vi "Update.vi"(8 "error in":errorcluster, 10 "object ref in":T1, 11 "Multi Column Listbox in":refnum<class "Multi Column Listbox.lvclass">) -> (0 "error out":errorcluster, 2 "object ref out":T1, 3 "Multi Column Listbox out":refnum<class "Multi Column Listbox.lvclass">)   [LabVIEW 2013, in "Table Manager.lvlib" / "Multi Column Listbox.lvclass"]
doc: "Updates the strings displayed in the MCLB."
uses:
  Multi Column Listbox.lvclass
  Table Manager/object ref.ctl
  Configuration Editor/Classes/Engine Parent/Engine Parent Editor Node.lvclass
  Configuration Editor/Classes/Module editor node/module editor node.lvclass
  Multi Column Listbox.lvclass/Multi Column Listbox.ctl
  Table Manager/Table Manager.lvclass/Table Manager.ctl
  Read Listbox.vi
  Table Manager/Read Index.vi
  Table Manager/Table Manager.lvclass
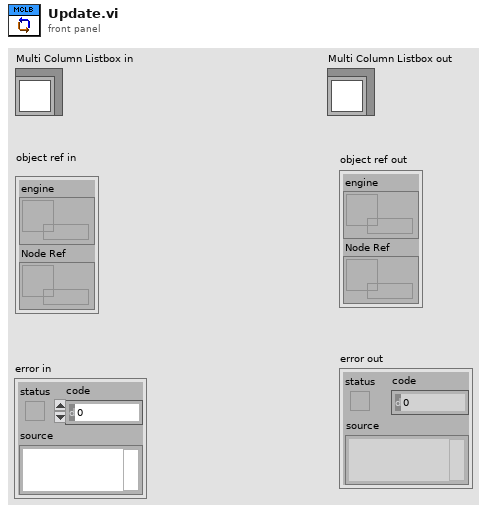
[diagram p1: front panel]
types:
  T1 = typedef "Table Manager.lvlib/Table Manager.lvclass/object ref.ctl" = cluster{"engine":refnum<data-value>, "Node Ref":refnum<data-value>}
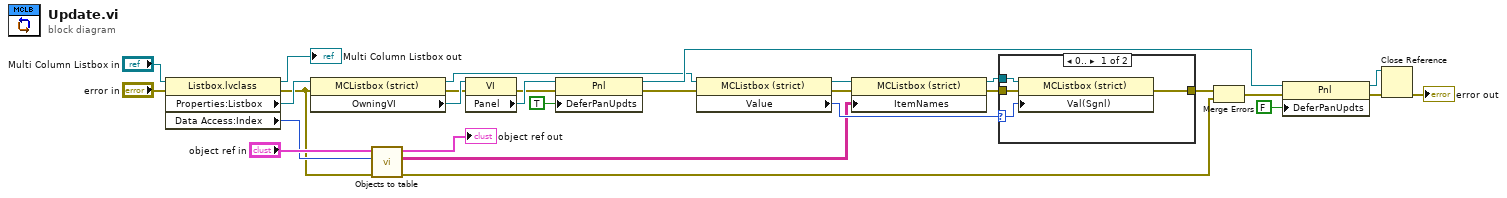
[diagram p0: block diagram]
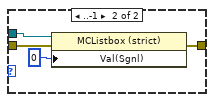
[diagram p2: hidden frame]
diagram:
  n1 = property class="Listbox.lvclass"(reference="Multi Column Listbox in", error in="error in") -> (reference out=→"Multi Column Listbox out":refnum<class "Multi Column Listbox.lvclass">, error out=w1:errorcluster, "Properties:Listbox"=w5:refnum<vi>, "Data Access:Index"=w6:i32)
  n2 = property class="MCListbox (strict)"(reference=w5, error in=w1) -> (reference out=w23:refnum<vi>, error out=w21:errorcluster, "OwningVI"=w22:refnum<vi>)
  n3 = call "Objects to table.vi"("error in (no error)"=w1, "Table Index"=w6, "object ref in"="object ref in") -> ("error out"=w9:errorcluster, "table"=w12:string[][], "object ref out"=→"object ref out":T1)  [unwired: 6 in]
  n4 = property class="VI"(reference=w22, error in=w21) -> (error out=w27:errorcluster, "Panel"=w28:refnum<vi>)  [unwired: 1 out]
  n5 = property class="Pnl"(reference=w28, error in=w27, "DeferPanUpdts"=TRUE ("Defer Panel Updates")) -> (reference out=w25:refnum<vi>, error out=w14:errorcluster)
  n6 = property class="MCListbox (strict)"(reference=w23, error in=w14) -> (reference out=w19:refnum<vi>, error out=w15:errorcluster, "Value"=w16:i32)
  n7 = property class="MCListbox (strict)"(reference=w19, error in=w15, "ItemNames"=w12) -> (reference out=w18:refnum<vi>, error out=w17:errorcluster)
  n8 = case shown="0.." w16 {
    selector: w16 -> [w30 _]
    tunnel: w18 -> [w33 w37]
    tunnel: w17 -> [w32 w36]
    tunnel: [w31 w35] -> w10
    frame 0.. {
      n9 = property class="MCListbox (strict)"(reference=w33, error in=w32, "Val(Sgnl)"=w30) -> (error out=w31:errorcluster)  [unwired: 1 out]
    }
    frame ..-1 {
      n10 = property class="MCListbox (strict)"(reference=w37, error in=w36, "Val(Sgnl)"=0 ("Value (Signaling)")) -> (error out=w35:errorcluster)  [unwired: 1 out]
    }
  }
  n11 = Merge Errors(w10, w9) -> (w8:errorcluster)
  n12 = property class="Pnl"(reference=w25, error in=w8, "DeferPanUpdts"=FALSE ("Defer Panel Updates")) -> (reference out=w20:refnum<vi>, error out=w24:errorcluster)
  n13 = Close Reference(reference=w20, error in (no error)=w24) -> (error out=→"error out":errorcluster)
